vi "Type Characters.vi"(9 "Length of Key Press (ms)":u32, 11 "Key Array":T1(array[cluster])) -> ()   [LabVIEW 2020, in "MacroAssert.lvlib"]
uses:
  MacroAssert.lvlib
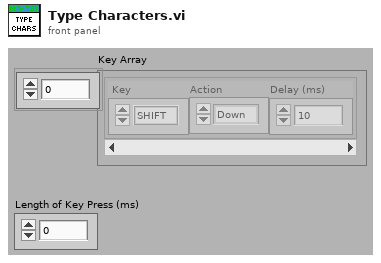
[diagram p1: front panel]
types:
  T1 = cluster{" Key":u8, "Action":enum16{"Press", "Up", "Down"}, "Delay (ms)":u32}[]
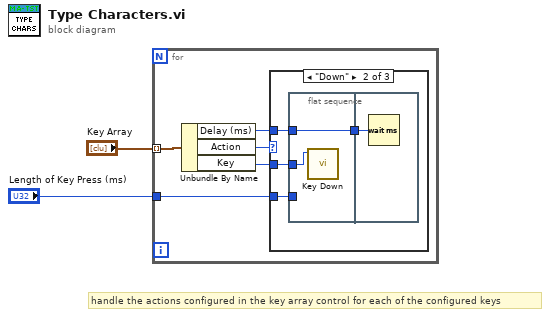
[diagram p0: block diagram]
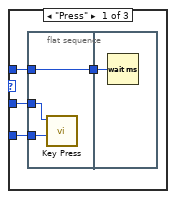
[diagram p2: hidden frame]
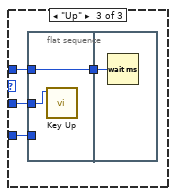
[diagram p3: hidden frame]
diagram:
  # "handle the actions configured in the key array control for each of the configured keys"
  n1 = for {
    tunnel: "Key Array" -> [w7] mode=indexing
    tunnel: "Length of Key Press (ms)" -> [w6]
    n2 = Unbundle By Name(w7) -> ("Delay (ms)"=w3:u32, "Action"=w5:enum16{"Press", "Up", "Down"}, "Key"=w4:u8)
    n3 = case shown="\"Down\"" w5 {
      tunnel: w6 -> [w11 w19 w26]
      tunnel: w4 -> [w10 w18 w25]
      tunnel: w3 -> [w8 w16 w23]
      frame "Press" {
        n4 = flat-sequence {
          tunnel: w11 -> [w14]
          tunnel: w10 -> [w13]
          tunnel: [w12] -> w9
          tunnel: w8 -> [w12]
          tunnel: w9 -> [w15]
          frame #0 {
            n5 = call "Key Press.vi"("ms wait after up (20)"=w14, "Virtual Key"=w13) -> ()  [unwired: 9 in, 1 out]
          }
          frame #1 {
            n6 = Wait (ms)(milliseconds to wait=w15) -> ()  [unwired: 1 out]
          }
        }
      }
      frame "Down" {
        n7 = flat-sequence {
          tunnel: w19 -> [_]
          tunnel: w18 -> [w20]
          tunnel: [w21] -> w17
          tunnel: w16 -> [w21]
          tunnel: w17 -> [w22]
          frame #0 {
            n8 = call "Key Down.vi"("Virtual Key"=w20) -> ()  [unwired: 10 in, 1 out]
          }
          frame #1 {
            n9 = Wait (ms)(milliseconds to wait=w22) -> ()  [unwired: 1 out]
          }
        }
      }
      frame "Up" {
        n10 = flat-sequence {
          tunnel: w26 -> [_]
          tunnel: w25 -> [w27]
          tunnel: [w28] -> w24
          tunnel: w23 -> [w28]
          tunnel: w24 -> [w29]
          frame #0 {
            n11 = call "Key Up.vi"("Virtual Key"=w27) -> ()  [unwired: 10 in, 1 out]
          }
          frame #1 {
            n12 = Wait (ms)(milliseconds to wait=w29) -> ()  [unwired: 1 out]
          }
        }
      }
    }
  }
